vi "WFDC Get XY Drift.vi"(0 "Ref Images":T1[](array[typedef]), 2 "Half Fit Box":i32, 5 "Current Image":u16[][](array[numeric]), 7 "CC Threshold":dbl, 9 "Roundness Ratio":dbl, 11 "Error In":errorcluster) -> (4 "Axis 1 Drift (px)":dbl, 6 "Axis 2 Drift (px)":dbl, 8 "CC Image":dbl[][](array[numeric]), 10 "CC Fit":dbl[][](array[numeric]), 15 "Error Out":errorcluster)   [LabVIEW 2020]
uses:
  <vilib>/vision/Image Controls.llb/IMAQ Image.ctl
panel:
  out "Half":i32
  in  "Size":i32
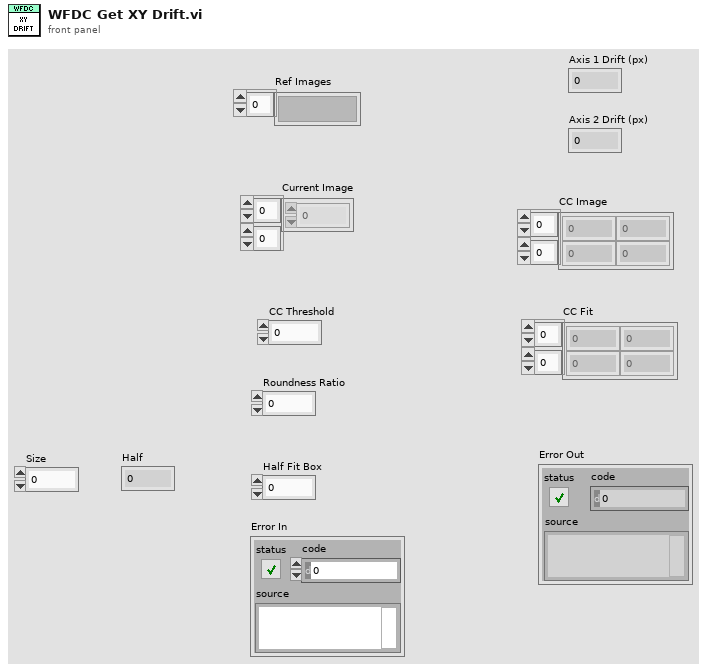
[diagram p1: front panel]
types:
  T1 = typedef "IMAQ Image.ctl" = refnum<image>
  T2 = typedef "2D Gaussian - Best Fit Parameters.ctl" = cluster{"Amplitude":dbl, "X Position":dbl, "Y Position":dbl, "X Width":dbl, "Y Width":dbl, "Offset":dbl}
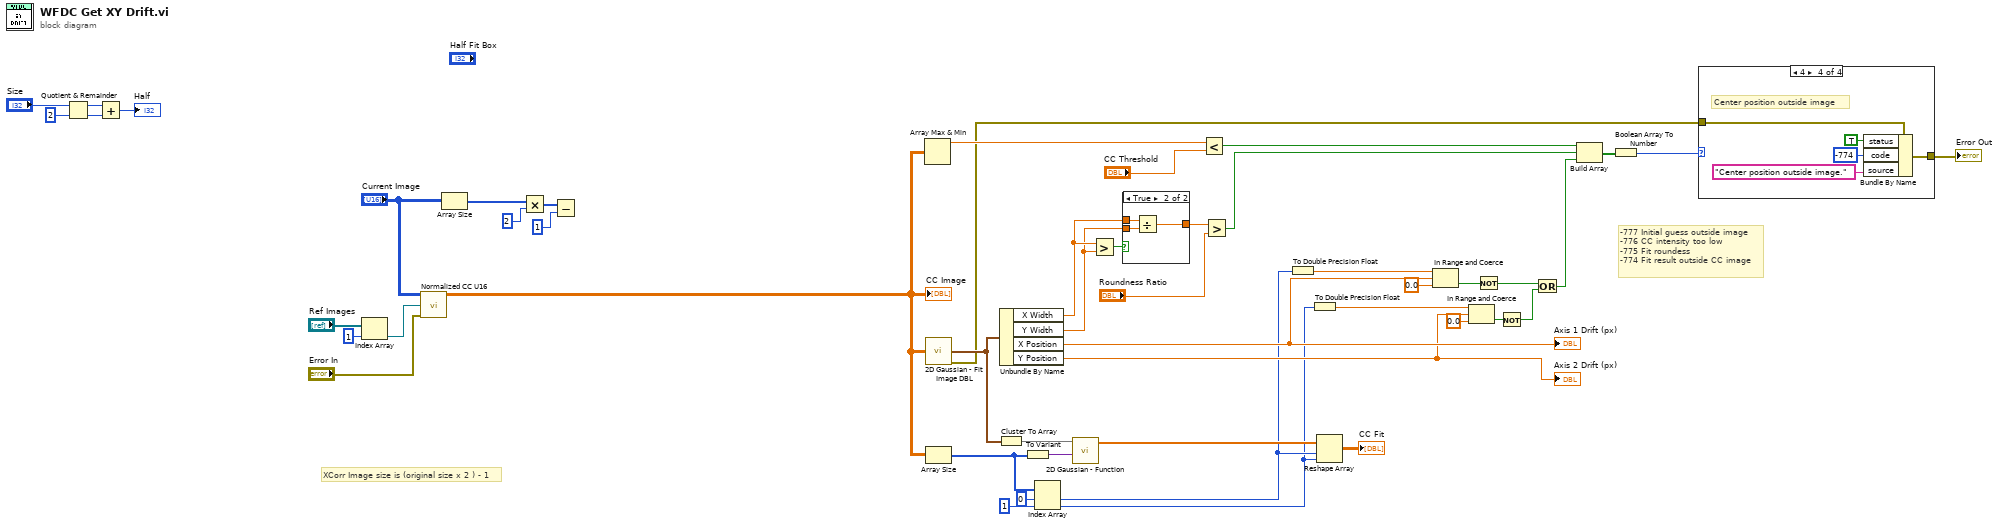
[diagram p0: block diagram]
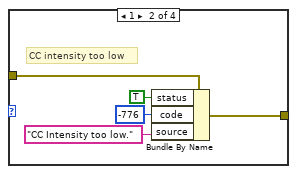
[diagram p3: hidden frame]
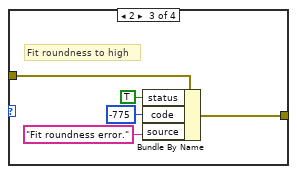
[diagram p4: hidden frame]
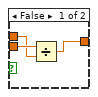
[diagram p5: hidden frame]
diagram:
  # "XCorr Image size is (original size x 2 ) - 1"
  # "-777 Initial guess outside image\n-776 CC intensity too low\n-775 Fit roundess\n-774 Fit result outside CC image"
  n1 = Quotient & Remainder(x="Size", y=2) -> (x-y*floor(x/y)=w2:i32, floor(x/y)=w3:i32)
  n2 = Add(x=w2, y=w3) -> (x+y=→"Half":i32)
  n3 = Index Array(array="Ref Images", index=1) -> (element=w15:T1)
  n4 = call "Normalized CC U16.vi"("Template U16"="Current Image", "A U16"=w15, "Error In"="Error In") -> ("normxcorr2"=w13:dbl[][])  [unwired: 10 in, 2 out]
  "CC Image" <- w13
  n5 = Array Size(array="Current Image") -> (size(s)=w9:i32[])
  n6 = Multiply(x=w9, y=2) -> (x*y=w7:i32[])
  n7 = Subtract(x=w7, y=1) -> ()  [unwired: 1 out]
  n8 = Array Max & Min(array=w13) -> (max value=w39:dbl)  [unwired: 3 out]
  n9 = call "2D Gaussian - Fit Image DBL.vi"("Image In (DBL)"=w13) -> ("Best Fit Params"=w47:T2, "Error Out"=w22:errorcluster)  [unwired: 13 in]
  n10 = Array Size(array=w13) -> (size(s)=w44:i32[])
  n11 = Cluster To Array(cluster=w47) -> (array=w42:dbl[])
  n12 = Unbundle By Name(w47) -> ("X Width"=w17:dbl, "Y Width"=w16:dbl, "X Position"=w37:dbl, "Y Position"=w36:dbl)
  "Axis 2 Drift (px)" <- w36
  "Axis 1 Drift (px)" <- w37
  n13 = To Variant(anything=w44) -> (Variant=w41:variant)
  n14 = Index Array(array=w44, index #1=0 ("index"), index #2=1 ("index")) -> (element #1=w20:i32, element #2=w19:i32)
  n15 = call "2D Gaussian - Function.vi"("data"=w41, "a"=w42) -> ("f(X,a)"=w43:dbl[])  [unwired: 2 in, 2 out]
  n16 = Greater?(x=w17, y=w16) -> (0:w31:bool)
  n17 = case shown="True" w31 {
    tunnel: w17 -> [w51 w55]
    tunnel: w16 -> [w52 w54]
    tunnel: [w50 w53] -> w30
    frame False {
      n18 = Divide(x=w52, y=w51) -> (x/y=w50:dbl)
    }
    frame True {
      n19 = Divide(x=w55, y=w54) -> (x/y=w53:dbl)
    }
  }
  n20 = Less?(x=w39, y="CC Threshold") -> (x < y?=w27:bool)
  n21 = Greater?(x=w30, y="Roundness Ratio") -> (0:w26:bool)
  n22 = To Double Precision Float(number=w20) -> (double precision float=w12:dbl)
  n23 = To Double Precision Float(number=w19) -> (double precision float=w11:dbl)
  n24 = Reshape Array(w43, w20, w19) -> (→"CC Fit":dbl[][])
  n25 = In Range and Coerce(upper limit=w12, x=w37, lower limit=0.0) -> (In Range?=w33:bool)  [unwired: 1 out]
  n26 = In Range and Coerce(upper limit=w11, x=w36, lower limit=0.0) -> (In Range?=w32:bool)  [unwired: 1 out]
  n27 = Not(x=w33) -> (.not. x?=w29:bool)
  n28 = Not(x=w32) -> (.not. x?=w28:bool)
  n29 = Or(x=w29, y=w28) -> (x .or. y?=w25:bool)
  n30 = Build Array(w27, w26, w25) -> (w24:bool[])
  n31 = Boolean Array To Number(Boolean array=w24) -> (number=w23:u32)
  n32 = case shown="4" w23 {
    tunnel: w22 -> [w56 w61 w63 w68]
    tunnel: [w56 w57 w62 w67] -> w21
    frame Default {
    }
    frame 1 {
      # "CC intensity too low"
      n33 = Bundle By Name(cluster=w61, "status"=TRUE, "code"=-776, "source"="CC Intensity too low.") -> (w57:errorcluster)
    }
    frame 2 {
      # "Fit roundness to high"
      n34 = Bundle By Name(cluster=w63, "status"=TRUE, "code"=-775, "source"="Fit roundness error.") -> (w62:errorcluster)
    }
    frame 4 {
      # "Center position outside image"
      n35 = Bundle By Name(cluster=w68, "status"=TRUE, "code"=-774, "source"="Center position outside image.") -> (w67:errorcluster)
    }
  }
  "Error Out" <- w21
